vi "FTW-Endpoint-Multipart-Receive.vi"(0 "FTW ØMQ Endpoint":refnum<class "FTW-Endpoint-ZMQ.lvclass">, 5 "Timeout":i32 format="%dmsec", 11 "error in":errorcluster) -> (4 "FTW ØMQ Endpoint out":refnum<class "FTW-Endpoint-ZMQ.lvclass">, 6 "Message Received":string[](array[string]), 8 "Timed out?":bool, 15 "error out":errorcluster)   [LabVIEW 2012, in "FTW-Endpoint-ZMQ.lvclass"]
uses:
  FTW-Endpoint-ZMQ.lvclass
  FTW-Endpoint-ZMQ.lvclass/FTW-Endpoint-ZMQ.ctl
panel:
  # "Inputs"
  # "Outputs"
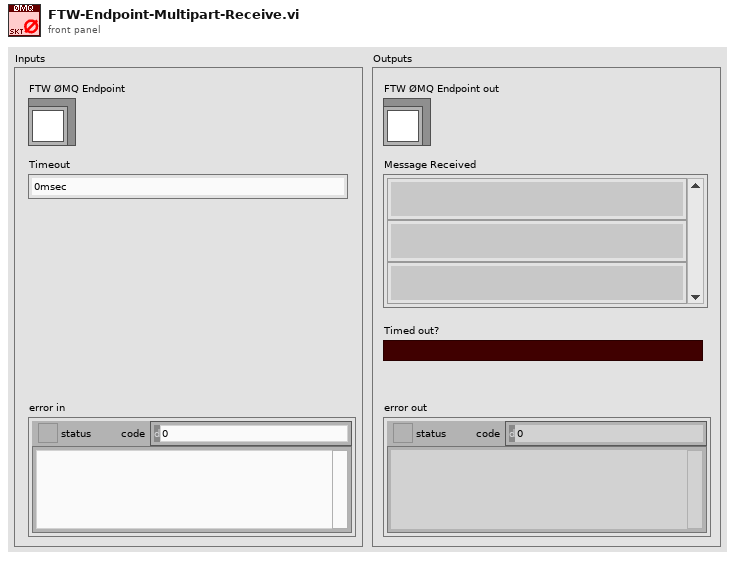
[diagram p1: front panel]
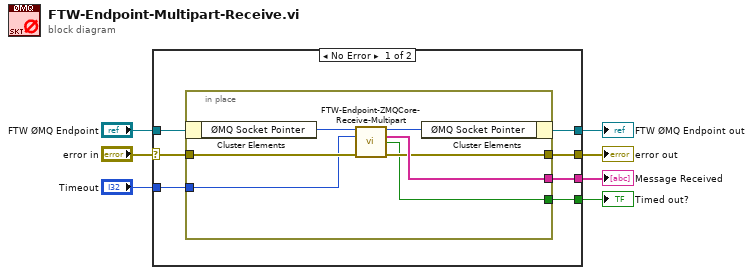
[diagram p0: block diagram]
diagram:
  n1 = case shown="No Error" "error in" {
    selector: "error in" -> [w12 w22]
    tunnel: "FTW ØMQ Endpoint" -> [w14 w23]
    tunnel: [w9 w22] -> w6
    tunnel: [w13 w23] -> w5
    tunnel: [w11 _] -> w3
    tunnel: "Timeout" -> [w10 _]
    tunnel: [w8 _] -> w1
    frame No Error {
      n2 = in-place {
        in-place-border: w12 -> [w21]
        in-place-border: [w18] -> w11
        in-place-border: w10 -> [w19]
        in-place-border: [w17] -> w9
        in-place-border: [w15] -> w8
        n3 = in-place-cluster #1(w14) -> ("ØMQ Socket Pointer"=w20:u64)
        n4 = call "FTW-Endpoint-ZMQCore-Receive-Multipart.vi"("ØMQ Socket Pointer"=w20, "Timeout"=w19, "error in"=w21) -> ("ØMQ Socket Pointer out"=w16:u64, "Multipart Message"=w18:string[], "Timed out?"=w15:bool, "error out"=w17:errorcluster)  [unwired: 9 in]
        n5 = in-place-cluster #1("ØMQ Socket Pointer"=w16) -> (w13:refnum<class "FTW-Endpoint-ZMQ.lvclass">)
      }
    }
    frame Error {
    }
  }
  "error out" <- w6
  "FTW ØMQ Endpoint out" <- w5
  "Message Received" <- w3
  "Timed out?" <- w1
